vi "VI Tree.vi"   [LabVIEW 2011, in "Agilent N432A.lvlib"]
doc: "This is the instrument driver for the <INSTRUMENT NAME>. The VI Tree displays all the user-callable VIs of the instrument driver in an organized table."
uses:
  <instrlib>/Agilent N432A/Agilent N432A.lvlib
panel:
  # "(c) 2007 <Enter Company Name Here>.  ALL RIGHTS RESERVED."
  # "SEE DIAGRAM\nFOR VI TREE."
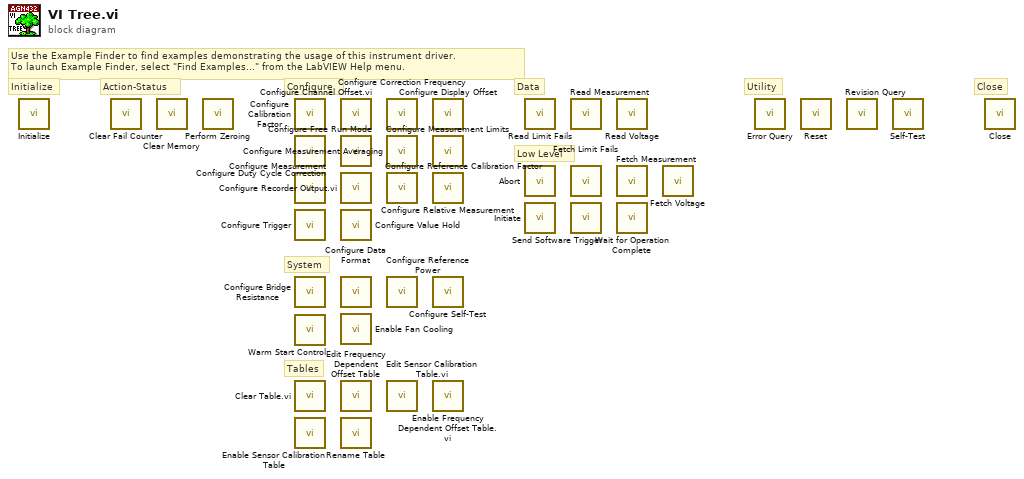
[diagram p0: block diagram]
diagram:
  # "Close"
  # "Utility"
  # "Low Level"
  # "Data"
  # "Tables"
  # "System"
  # "Configure"
  # "Action-Status"
  # "Initialize"
  # "Use the Example Finder to find examples demonstrating the usage of this instrument driver.\nTo launch Example Finder, select \"Find Examples...\" from the LabVIEW Help menu."
  n1 = call <instrlib>:"Initialize.vi"() -> ()  [unwired: 10 in, 2 out]
  n2 = call <instrlib>:"Clear Fail Counter.vi"() -> ()  [unwired: 10 in, 2 out]
  n3 = call <instrlib>:"Clear Memory.vi"() -> ()  [unwired: 10 in, 2 out]
  n4 = call <instrlib>:"Perform Zeroing.vi"() -> ()  [unwired: 10 in, 2 out]
  n5 = call <instrlib>:"Configure Calibration Factor.vi"() -> ()  [unwired: 10 in, 2 out]
  n6 = call <instrlib>:"Configure Duty Cycle Correction.vi"() -> ()  [unwired: 10 in, 2 out]
  n7 = call <instrlib>:"Configure Measurement.vi"() -> ()  [unwired: 10 in, 2 out]
  n8 = call <instrlib>:"Configure Trigger.vi"() -> ()  [unwired: 10 in, 2 out]
  n9 = call <instrlib>:"Configure Bridge Resistance.vi"() -> ()  [unwired: 10 in, 2 out]
  n10 = call <instrlib>:"Warm Start Control.vi"() -> ()  [unwired: 10 in, 2 out]
  n11 = call <instrlib>:"Clear Table.vi.vi"() -> ()  [unwired: 10 in, 2 out]
  n12 = call <instrlib>:"Enable Sensor Calibration Table.vi"() -> ()  [unwired: 10 in, 2 out]
  n13 = call <instrlib>:"Configure Channel Offset.vi.vi"() -> ()  [unwired: 10 in, 2 out]
  n14 = call <instrlib>:"Configure Free Run Mode.vi"() -> ()  [unwired: 10 in, 2 out]
  n15 = call <instrlib>:"Configure Recorder Output.vi.vi"() -> ()  [unwired: 10 in, 2 out]
  n16 = call <instrlib>:"Configure Value Hold.vi"() -> ()  [unwired: 10 in, 2 out]
  n17 = call <instrlib>:"Configure Data Format.vi"() -> ()  [unwired: 10 in, 2 out]
  n18 = call <instrlib>:"Enable Fan Cooling.vi"() -> ()  [unwired: 10 in, 2 out]
  n19 = call <instrlib>:"Edit Frequency Dependent Offset Table.vi"() -> ()  [unwired: 10 in, 2 out]
  n20 = call <instrlib>:"Rename Table.vi"() -> ()  [unwired: 10 in, 2 out]
  n21 = call <instrlib>:"Configure Correction Frequency.vi"() -> ()  [unwired: 10 in, 2 out]
  n22 = call <instrlib>:"Configure Measurement Averaging.vi"() -> ()  [unwired: 10 in, 2 out]
  n23 = call <instrlib>:"Configure Reference Calibration Factor.vi"() -> ()  [unwired: 10 in, 2 out]
  n24 = call <instrlib>:"Configure Reference Power.vi"() -> ()  [unwired: 10 in, 2 out]
  n25 = call <instrlib>:"Edit Sensor Calibration Table.vi.vi"() -> ()  [unwired: 10 in, 2 out]
  n26 = call <instrlib>:"Configure Display Offset.vi"() -> ()  [unwired: 10 in, 2 out]
  n27 = call <instrlib>:"Configure Measurement Limits.vi"() -> ()  [unwired: 10 in, 2 out]
  n28 = call <instrlib>:"Configure Relative Measurement.vi"() -> ()  [unwired: 10 in, 2 out]
  n29 = call <instrlib>:"Configure Self-Test.vi"() -> ()  [unwired: 10 in, 2 out]
  n30 = call <instrlib>:"Enable Frequency Dependent Offset Table.vi.vi"() -> ()  [unwired: 10 in, 2 out]
  n31 = call <instrlib>:"Read Limit Fails.vi"() -> ()  [unwired: 8 in, 4 out]
  n32 = call <instrlib>:"Abort.vi"() -> ()  [unwired: 10 in, 2 out]
  n33 = call <instrlib>:"Initiate.vi"() -> ()  [unwired: 10 in, 2 out]
  n34 = call <instrlib>:"Read Measurement.vi"() -> ()  [unwired: 9 in, 3 out]
  n35 = call <instrlib>:"Fetch Limit Fails.vi"() -> ()  [unwired: 8 in, 4 out]
  n36 = call <instrlib>:"Send Software Trigger.vi"() -> ()  [unwired: 10 in, 2 out]
  n37 = call <instrlib>:"Read Voltage.vi"() -> ()  [unwired: 10 in, 2 out]
  n38 = call <instrlib>:"Fetch Measurement.vi"() -> ()  [unwired: 9 in, 3 out]
  n39 = call <instrlib>:"Wait for Operation Complete.vi"() -> ()  [unwired: 10 in, 2 out]
  n40 = call <instrlib>:"Fetch Voltage.vi"() -> ()  [unwired: 9 in, 3 out]
  n41 = call <instrlib>:"Error Query.vi"() -> ()  [unwired: 8 in, 4 out]
  n42 = call <instrlib>:"Reset.vi"() -> ()  [unwired: 10 in, 2 out]
  n43 = call <instrlib>:"Revision Query.vi"() -> ()  [unwired: 8 in, 4 out]
  n44 = call <instrlib>:"Self-Test.vi"() -> ()  [unwired: 8 in, 4 out]
  n45 = call <instrlib>:"Close.vi"() -> ()  [unwired: 11 in, 1 out]
